vi "Get SMO Serial Number.vi"(8 "error in (no error)":errorcluster, 11 "Instrument.Framework-Template in":refnum<class "Instrument.Framework-Template.lvclass">) -> (0 "error out":errorcluster, 2 "Serial Number":string, 3 "Instrument.Framework-Template out":refnum<class "Instrument.Framework-Template.lvclass">)   [LabVIEW 2019, in "Instrument.Framework-Template.lvclass"]
doc: "Override this VI to return the port number of your Instrument"
uses:
  Instrument.Framework-Template.lvclass
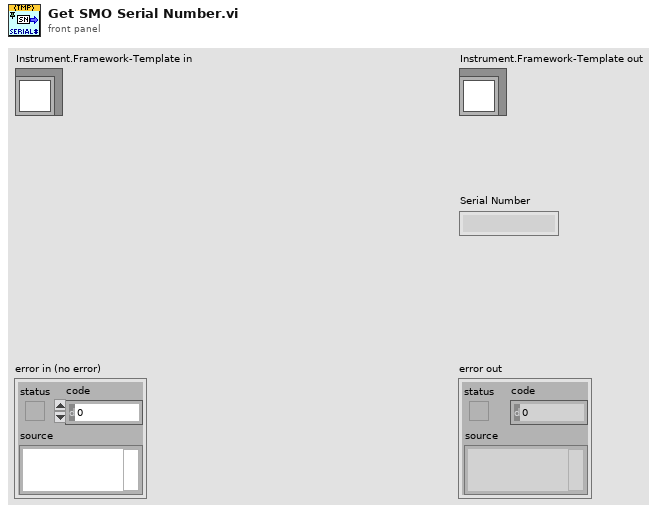
[diagram p1: front panel]
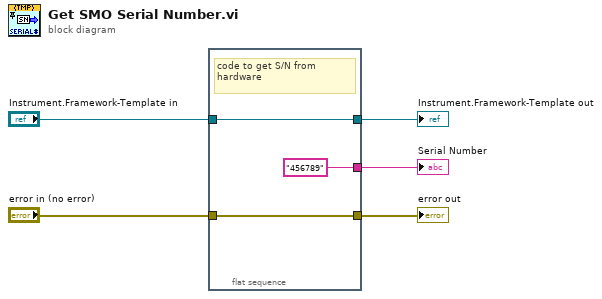
[diagram p0: block diagram]
diagram:
  n1 = flat-sequence {
    tunnel: "Instrument.Framework-Template in" -> [w8]
    tunnel: [w8] -> w4
    tunnel: [w7] -> w3
    tunnel: "error in (no error)" -> [w7]
    tunnel: ["456789" ("Serial Number")] -> w1
    frame #0 {
      # "code to get S/N from hardware"
    }
  }
  "error out" <- w3
  "Instrument.Framework-Template out" <- w4
  "Serial Number" <- w1
